vi "Read SPI_FRM_Array.vi"(8 "error in (no error)":errorcluster, 11 "Config_Read_SPI in":refnum<class "Config_Read_SPI.lvclass">) -> (0 "error out":errorcluster, 2 "SPI_FRM_Array":T1[](array[typedef]) {"Addr" format="%x"; "Data" format="%x"}, 3 "Config_Read_SPI out":refnum<class "Config_Read_SPI.lvclass">)   [LabVIEW 2018, in "Config_Read_SPI.lvclass"]
uses:
  Config_Read_SPI.lvclass
  SPI_FRM_Config.ctl
  Classes/Config_Read/RW_Option.ctl
  SPI_Mode.ctl
  Config_Read_SPI.lvclass/Config_Read_SPI.ctl
  Classes/Config_Read/Config_Read_BML.lvclass
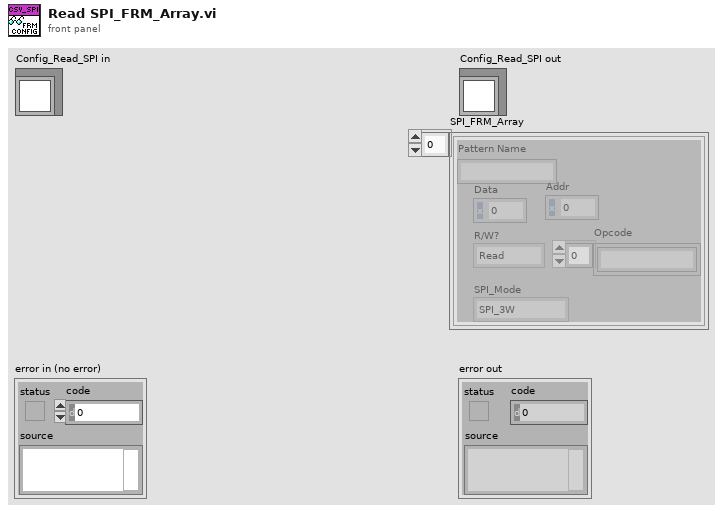
[diagram p1: front panel]
types:
  T1 = typedef "Config_Read_SPI.lvclass/SPI_FRM_Config.ctl" = cluster{"Pattern Name":string, "Data":u16, "Addr":u16, "R/W?":T2, "Opcode":string[], "SPI_Mode":T3}
  T2 = typedef "Config_Read_BML.lvclass/RW_Option.ctl" = enum16{"Read", "Write", "R/W"}
  T3 = typedef "Config_Read_SPI.lvclass/SPI_Mode.ctl" = enum16{"SPI_3W", "SPI_4W"}
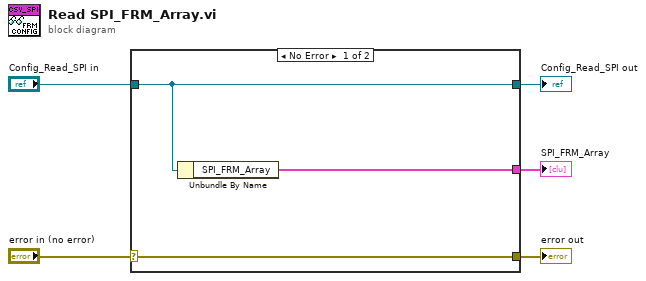
[diagram p0: block diagram]
diagram:
  n1 = case shown="No Error" "error in (no error)" {
    selector: "error in (no error)" -> [w8 w9]
    tunnel: [w8 w9] -> w4
    tunnel: [w7 w10] -> w2
    tunnel: "Config_Read_SPI in" -> [w7 w10]
    tunnel: [w6 _] -> w1
    frame No Error {
      n2 = Unbundle By Name(w7) -> ("SPI_FRM_Array"=w6:T1[])
    }
    frame Error {
    }
  }
  "error out" <- w4
  "Config_Read_SPI out" <- w2
  "SPI_FRM_Array" <- w1
